vi "initial_event.vi"   [LabVIEW 2016]
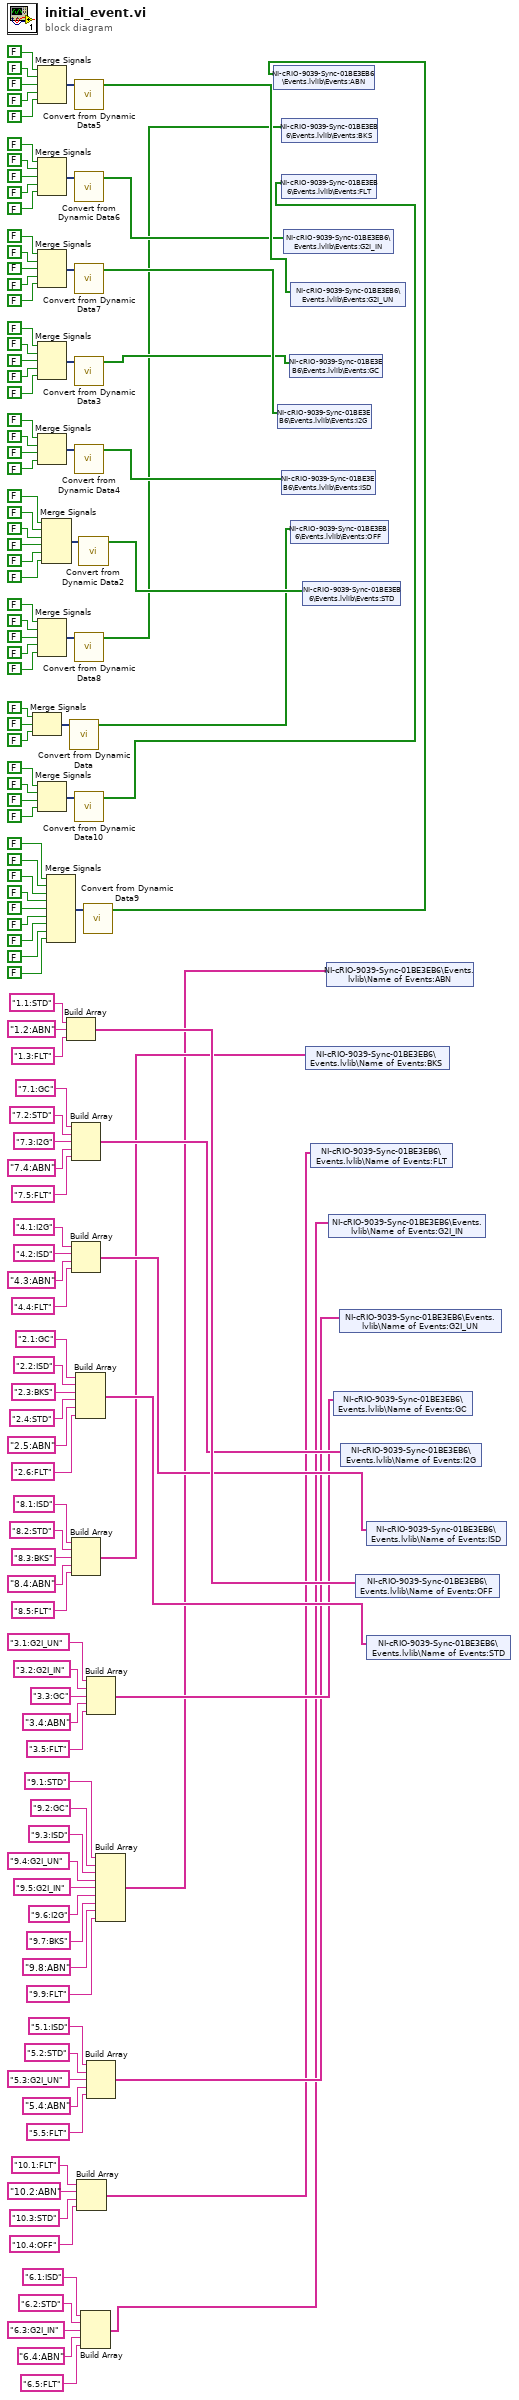
[diagram p0: block diagram]
diagram:
  n1 = Merge Signals(FALSE, FALSE, FALSE) -> (w132:dynamicdata)
  n2 = Merge Signals(FALSE, FALSE, FALSE, FALSE, FALSE) -> (w92:dynamicdata)
  n3 = Merge Signals(FALSE, FALSE, FALSE, FALSE, FALSE) -> (w86:dynamicdata)
  n4 = Merge Signals(FALSE, FALSE, FALSE, FALSE, FALSE) -> (w80:dynamicdata)
  n5 = Merge Signals(FALSE, FALSE, FALSE, FALSE, FALSE) -> (w112:dynamicdata)
  n6 = Merge Signals(FALSE, FALSE, FALSE, FALSE) -> (w101:dynamicdata)
  n7 = Merge Signals(FALSE, FALSE, FALSE, FALSE, FALSE) -> (w74:dynamicdata)
  n8 = Merge Signals(FALSE, FALSE, FALSE, FALSE) -> (w58:dynamicdata)
  n9 = Merge Signals(FALSE, FALSE, FALSE, FALSE, FALSE, FALSE) -> (w125:dynamicdata)
  n10 = Merge Signals(FALSE, FALSE, FALSE, FALSE, FALSE, FALSE, FALSE, FALSE, FALSE) -> (w68:dynamicdata)
  n11 = Build Array("1.1:STD", "1.2:ABN", "1.3:FLT") -> (w10:string[])
  n12 = call "Convert from Dynamic Data"("Dynamic Data Type"=w132) -> ("Array"=w13:bool[])  [unwired: 3 in]
  n13 = Build Array("7.1:GC", "7.2:STD", "7.3:I2G", "7.4:ABN", "7.5:FLT") -> (w9:string[])
  n14 = Build Array("4.1:I2G", "4.2:ISD", "4.3:ABN", "4.4:FLT") -> (w8:string[])
  n15 = Build Array("8.1:ISD", "8.2:STD", "8.3:BKS", "8.4:ABN", "8.5:FLT") -> (w6:string[])
  n16 = call "Convert from Dynamic Data5"("Dynamic Data Type"=w92) -> ("Array"=w20:bool[])  [unwired: 3 in]
  n17 = call "Convert from Dynamic Data6"("Dynamic Data Type"=w86) -> ("Array"=w19:bool[])  [unwired: 3 in]
  n18 = call "Convert from Dynamic Data7"("Dynamic Data Type"=w80) -> ("Array"=w18:bool[])  [unwired: 3 in]
  n19 = call "Convert from Dynamic Data3"("Dynamic Data Type"=w112) -> ("Array"=w17:bool[])  [unwired: 3 in]
  n20 = call "Convert from Dynamic Data4"("Dynamic Data Type"=w101) -> ("Array"=w16:bool[])  [unwired: 3 in]
  n21 = call "Convert from Dynamic Data8"("Dynamic Data Type"=w74) -> ("Array"=w14:bool[])  [unwired: 3 in]
  n22 = call "Convert from Dynamic Data10"("Dynamic Data Type"=w58) -> ("Array"=w12:bool[])  [unwired: 3 in]
  n23 = Build Array("2.1:GC", "2.2:ISD", "2.3:BKS", "2.4:STD", "2.5:ABN", "2.6:FLT") -> (w7:string[])
  n24 = Build Array("10.1:FLT", "10.2:ABN", "10.3:STD", "10.4:OFF") -> (w2:string[])
  n25 = call "Convert from Dynamic Data2"("Dynamic Data Type"=w125) -> ("Array"=w15:bool[])  [unwired: 3 in]
  n26 = Build Array("6.1:ISD", "6.2:STD", "6.3:G2I_IN", "6.4:ABN", "6.5:FLT") -> (w1:string[])
  n27 = call "Convert from Dynamic Data9"("Dynamic Data Type"=w68) -> ("Array"=w11:bool[])  [unwired: 3 in]
  n28 = Build Array("3.1:G2I_UN", "3.2:G2I_IN", "3.3:GC", "3.4:ABN", "3.5:FLT") -> (w5:string[])
  n29 = Build Array("5.1:ISD", "5.2:STD", "5.3:G2I_UN", "5.4:ABN", "5.5:FLT") -> (w3:string[])
  n30 = Build Array("9.1:STD", "9.2:GC", "9.3:ISD", "9.4:G2I_UN", "9.5:G2I_IN", "9.6:I2G", "9.7:BKS", "9.8:ABN", "9.9:FLT") -> (w4:string[])
  n31 = shared-variable "NI-cRIO-9039-Sync-01BE3EB6\\Events.lvlib\\Events:ABN"(w11) -> ()  [unwired: 1 in, 1 out]
  n32 = shared-variable "NI-cRIO-9039-Sync-01BE3EB6\\Events.lvlib\\Events:I2G"(w18) -> ()  [unwired: 1 in, 1 out]
  n33 = shared-variable "NI-cRIO-9039-Sync-01BE3EB6\\Events.lvlib\\Events:BKS"(w14) -> ()  [unwired: 1 in, 1 out]
  n34 = shared-variable "NI-cRIO-9039-Sync-01BE3EB6\\Events.lvlib\\Events:FLT"(w12) -> ()  [unwired: 1 in, 1 out]
  n35 = shared-variable "NI-cRIO-9039-Sync-01BE3EB6\\Events.lvlib\\Events:ISD"(w16) -> ()  [unwired: 1 in, 1 out]
  n36 = shared-variable "NI-cRIO-9039-Sync-01BE3EB6\\Events.lvlib\\Events:G2I_IN"(w19) -> ()  [unwired: 1 in, 1 out]
  n37 = shared-variable "NI-cRIO-9039-Sync-01BE3EB6\\Events.lvlib\\Events:GC"(w17) -> ()  [unwired: 1 in, 1 out]
  n38 = shared-variable "NI-cRIO-9039-Sync-01BE3EB6\\Events.lvlib\\Events:G2I_UN"(w20) -> ()  [unwired: 1 in, 1 out]
  n39 = shared-variable "NI-cRIO-9039-Sync-01BE3EB6\\Events.lvlib\\Events:OFF"(w13) -> ()  [unwired: 1 in, 1 out]
  n40 = shared-variable "NI-cRIO-9039-Sync-01BE3EB6\\Events.lvlib\\Events:STD"(w15) -> ()  [unwired: 1 in, 1 out]
  n41 = shared-variable "NI-cRIO-9039-Sync-01BE3EB6\\Events.lvlib\\Name of Events:BKS"(w6) -> ()  [unwired: 1 in, 1 out]
  n42 = shared-variable "NI-cRIO-9039-Sync-01BE3EB6\\Events.lvlib\\Name of Events:FLT"(w2) -> ()  [unwired: 1 in, 1 out]
  n43 = shared-variable "NI-cRIO-9039-Sync-01BE3EB6\\Events.lvlib\\Name of Events:ABN"(w4) -> ()  [unwired: 1 in, 1 out]
  n44 = shared-variable "NI-cRIO-9039-Sync-01BE3EB6\\Events.lvlib\\Name of Events:G2I_IN"(w1) -> ()  [unwired: 1 in, 1 out]
  n45 = shared-variable "NI-cRIO-9039-Sync-01BE3EB6\\Events.lvlib\\Name of Events:GC"(w5) -> ()  [unwired: 1 in, 1 out]
  n46 = shared-variable "NI-cRIO-9039-Sync-01BE3EB6\\Events.lvlib\\Name of Events:G2I_UN"(w3) -> ()  [unwired: 1 in, 1 out]
  n47 = shared-variable "NI-cRIO-9039-Sync-01BE3EB6\\Events.lvlib\\Name of Events:I2G"(w9) -> ()  [unwired: 1 in, 1 out]
  n48 = shared-variable "NI-cRIO-9039-Sync-01BE3EB6\\Events.lvlib\\Name of Events:OFF"(w10) -> ()  [unwired: 1 in, 1 out]
  n49 = shared-variable "NI-cRIO-9039-Sync-01BE3EB6\\Events.lvlib\\Name of Events:ISD"(w8) -> ()  [unwired: 1 in, 1 out]
  n50 = shared-variable "NI-cRIO-9039-Sync-01BE3EB6\\Events.lvlib\\Name of Events:STD"(w7) -> ()  [unwired: 1 in, 1 out]
